vi "Eye Diagram TODO.vi"() -> ()   [LabVIEW 2013]
uses:
  <vilib>/Analysis/2dsp.llb/1D Convolution (DBL).vi
  <vilib>/Analysis/NI_AALPro.lvlib
panel:
  out "Size":i32
  out "Sub Array":i32[](array[numeric])
  in  "Bit":i32[](array[numeric])=[0, 0, 0, 1, 0, 1, 1, 1, 0, 0]
  in  "Shaping Function":enum16{"Triangle", "Sinc", "Rcosine"}(ring)=enum."Sinc"
  out "Pattern":dbl[](graph)
  out "Eye Diagram":dbl[][](graph)
  # "Eye Diagram"
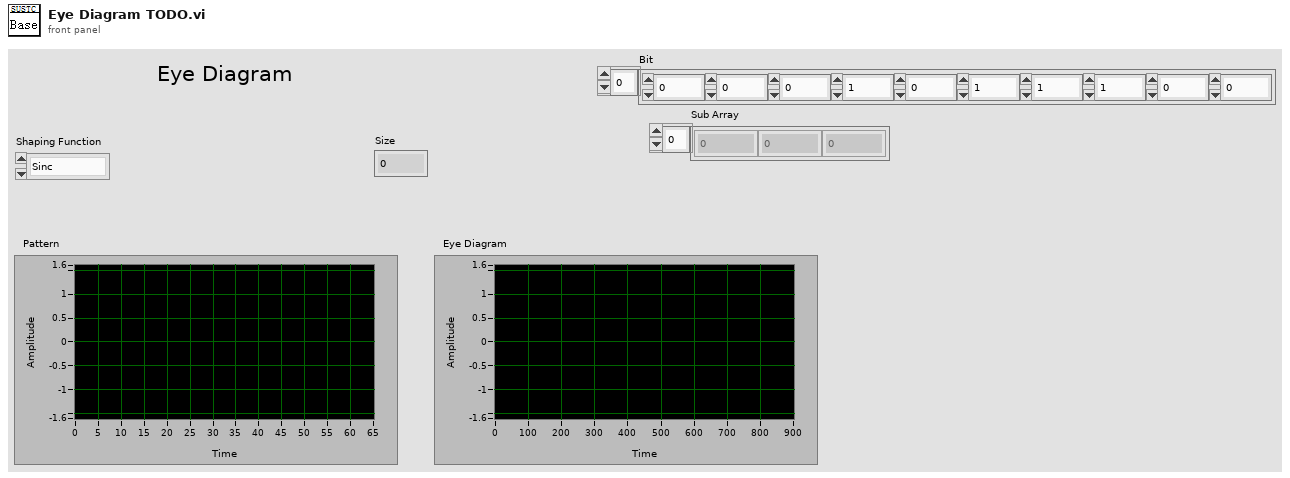
[diagram p1: front panel]
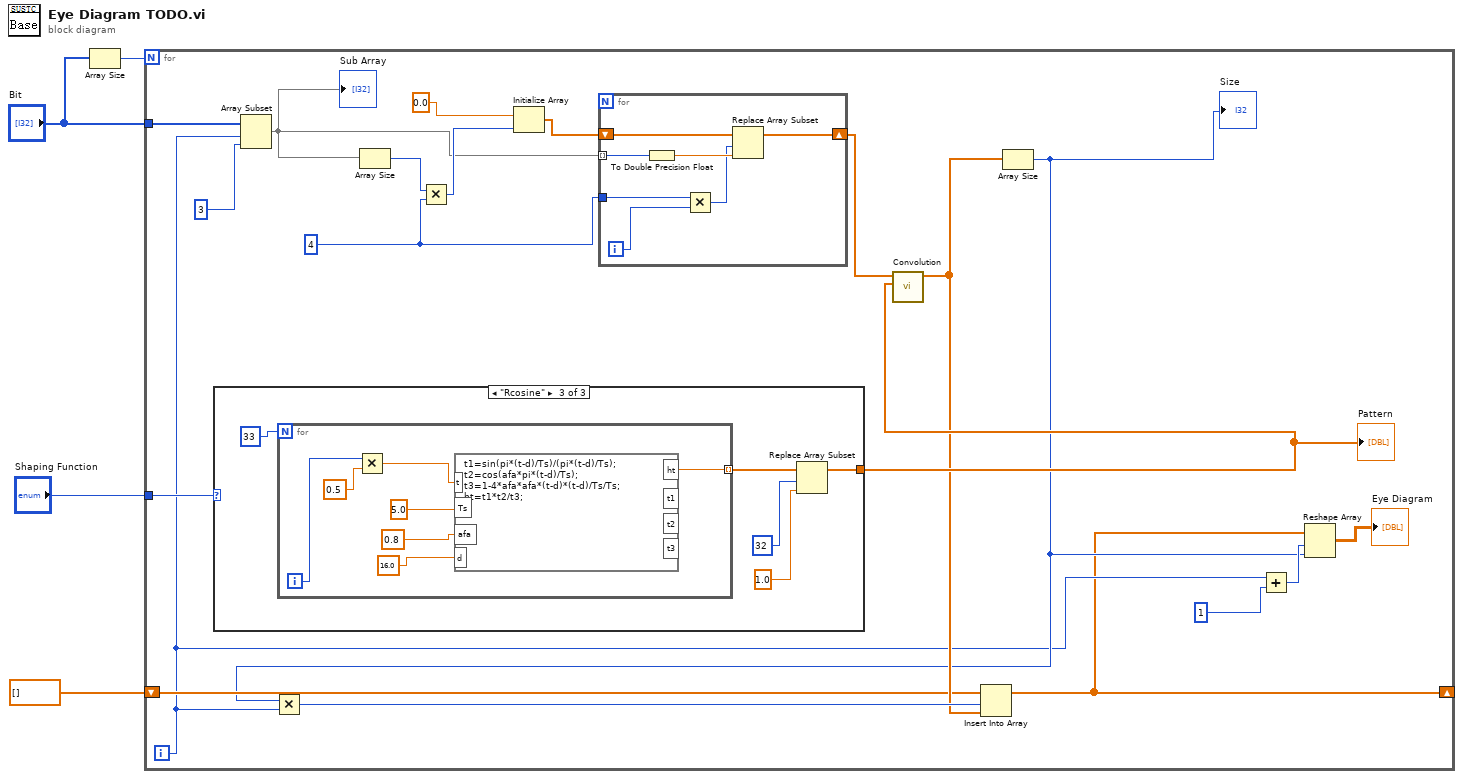
[diagram p0: block diagram]
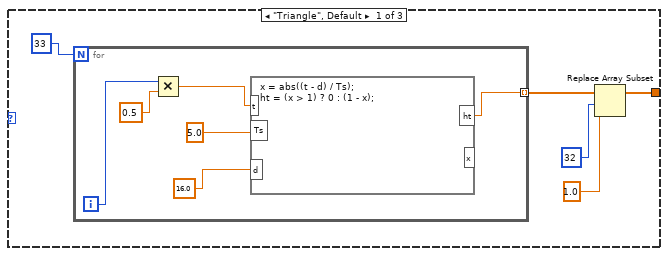
[diagram p2: hidden frame]
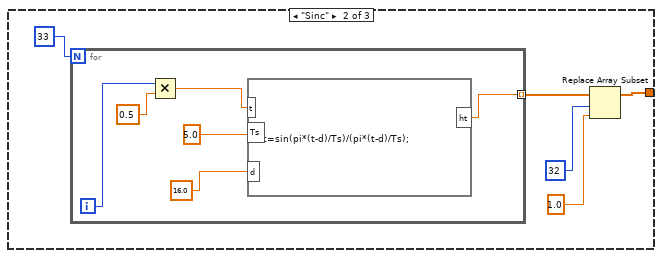
[diagram p3: hidden frame]
diagram:
  n1 = Array Size(array="Bit") -> (size(s)=w3:i32)
  n2 = for {
    N: w3 -> [_]
    tunnel: "Bit" -> [w21]
    tunnel: "Shaping Function" -> [w24]
    shift-right: [w5] -> _
    shift-left: dbl[] [] -> [w11]
    i -> [w6]
    w15 = 4
    n3 = case shown="\"Rcosine\"" w24 {
      tunnel: [w26 w38 w48] -> w23
      frame "Triangle", Default {
        n4 = for {
          N: 33 -> [_]
          tunnel: [w33] -> w27 mode=indexing
          i -> [w35]
          n5 = Multiply(x=w35, y=0.5) -> (x*y=w32:dbl)
          n6 = formula code="x = abs((t - d) / Ts);\nht = (x > 1) ? 0 : (1 - x);"("t"=w32, "Ts"=5.0, "d"=16.0) -> ("ht"=w33:dbl)  [unwired: 1 out]
        }
        n7 = Replace Array Subset(array=w27, new element=1.0, index=32) -> (w26:dbl[])
      }
      frame "Sinc" {
        n8 = for {
          N: 33 -> [_]
          tunnel: [w44] -> w37 mode=indexing
          i -> [w46]
          n9 = Multiply(x=w46, y=0.5) -> (x*y=w43:dbl)
          n10 = formula code="ht=sin(pi*(t-d)/Ts)/(pi*(t-d)/Ts);"("t"=w43, "Ts"=5.0, "d"=16.0) -> ("ht"=w44:dbl)
        }
        n11 = Replace Array Subset(array=w37, new element=1.0, index=32) -> (w38:dbl[])
      }
      frame "Rcosine" {
        n12 = for {
          N: 33 -> [_]
          tunnel: [w56] -> w49 mode=indexing
          i -> [w58]
          n13 = Multiply(x=w58, y=0.5) -> (x*y=w55:dbl)
          n14 = formula code="t1=sin(pi*(t-d)/Ts)/(pi*(t-d)/Ts);\nt2=cos(afa*pi*(t-d)/Ts);\nt3=1-4*afa*afa*(t-d)*(t-d)/Ts/Ts;\nht=t1*t2/t3;"("t"=w55, "Ts"=5.0, "d"=16.0, "afa"=0.8) -> ("ht"=w56:dbl)  [unwired: 3 out]
        }
        n15 = Replace Array Subset(array=w49, new element=1.0, index=32) -> (w48:dbl[])
      }
    }
    "Pattern" <- w23
    n16 = Array Subset(array=w21, index=w6, length=3) -> (w16:i32[])
    "Sub Array" <- w16
    n17 = Array Size(array=w16) -> (size(s)=w20:i32)
    n18 = Multiply(x=w20, y=w15) -> (x*y=w19:i32)
    n19 = Initialize Array(0.0, w19) -> (w17:dbl[])
    n20 = for {
      shift-right: [w64] -> w14
      shift-left: w17 -> [w65]
      tunnel: w16 -> [w62] mode=indexing
      tunnel: w15 -> [w61]
      i -> [w60]
      n21 = To Double Precision Float(number=w62) -> (double precision float=w63:dbl)
      n22 = Multiply(x=w61, y=w60) -> (x*y=w59:i32)
      n23 = Replace Array Subset(array=w65, new element=w63, index=w59) -> (w64:dbl[])
    }
    n24 = call-poly <vilib>:"Convolution.vi"("Y"=w23, "X"=w14) -> ("X * Y"=w12:dbl[])  [unwired: 8 in, 1 out]
    n25 = Array Size(array=w12) -> (size(s)=w7:i32)
    "Size" <- w7
    n26 = Multiply(x=w7, y=w6) -> (x*y=w13:i32)
    n27 = Insert Into Array(array=w11, index=w13, new element=w12) -> (w5:dbl[])
    n28 = Add(x=w6, y=1) -> (x+y=w8:i32)
    n29 = Reshape Array(w5, w8, w7) -> (→"Eye Diagram":dbl[][])
  }
